vi "tryRead.vi"(8 "error in (no error)":errorcluster, 11 "M1M3SAL in":refnum<class "M1M3SAL.lvclass">) -> (0 "error out":errorcluster, 1 "Timeout":bool, 2 "Message":T1, 3 "M1M3SAL out":refnum<class "M1M3SAL.lvclass">)   [LabVIEW 2016, in "M1M3SupportCommunicator.lvlib" / "M1M3SAL.lvclass"]
uses:
  M1M3SAL.lvclass
  DataTypes/Message.ctl
  DataTypes/MessageHeader.ctl
  DataTypes/MessageTypes.ctl
  DataTypes/MessageTopics.ctl
  M1M3SupportCommunicator.lvlib
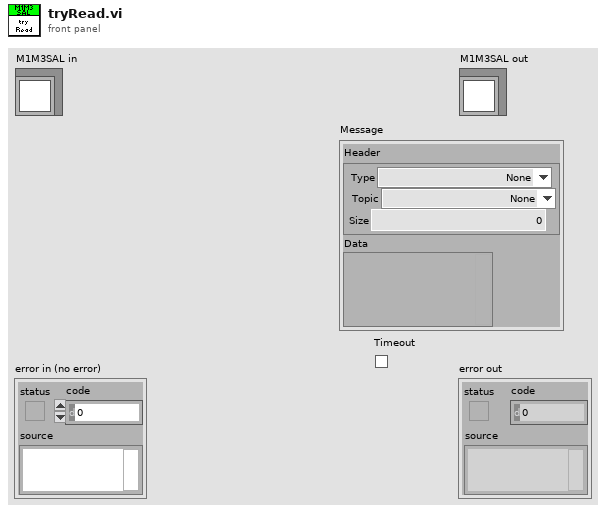
[diagram p1: front panel]
types:
  T1 = typedef "M1M3SupportCommunicator.lvlib/Message.ctl" = cluster{"Header":T2, "Data":variant}
  T2 = typedef "M1M3SupportCommunicator.lvlib/MessageHeader.ctl" = cluster{"Type":T3, "Topic":T4, "Size":i32}
  T3 = typedef "M1M3SupportCommunicator.lvlib/MessageTypes.ctl" = enum8{"None", "PutSample", "GetNextSample", "LogEvent", "GetEvent", "IssueCommand", "CommandId", "WaitForCompletion", "AcceptCommand", "AckCommand"}
  T4 = typedef "M1M3SupportCommunicator.lvlib/MessageTopics.ctl" = enum8{"None", "ForceActuatorData", "MirrorForceData", "HardpointData", "AirData", "DynamicData", "FPGAData", "IMSData", "ForceActuatorStatus", "ElevationData", "HardpointStatus", "HardpointActuatorChase", "AirStatus", "ForceActuatorSafetyChecks", "ForceActuatorTest", "ActuatorBroadcastCounter", "StatusChecks", "CellChecks", "HardpointActuatorBreakaway", "RaiseMirrorComplete", "ILCCommunication", "ElevationAngleChecks", "DetailedState", "ServoLoops", "ForceActuatorInfo", "LowerMirrorComplete", "HardpointActuatorInfo", "SettingsApplied", "ErrorCode", "StartupChecks", "SummaryState", "SettingVersions", "ActuatorTestStatus", "AppliedSettingsMatchStart", "Enable", "EnterMaintenance", "Standby", "AbortLowerM1M3", "ApplyAberrationByForces", "ApplyAOSCorrectionByBendingModes", "ClearAOSCorrection", "Start", "RaiseM1M3", "TestForceActuator", "LowerM1M3", "ApplyAOSCorrectionByForces", "Disable", "ApplyAberationByBendingMode", "TestHardpoint", "ManipulateM1M3", "ClearAberration", "Exit", "TestAir", "AbortRaiseM1M3", "MoveHardpointActuators", "ExitMaintenance", "Shutdown"}
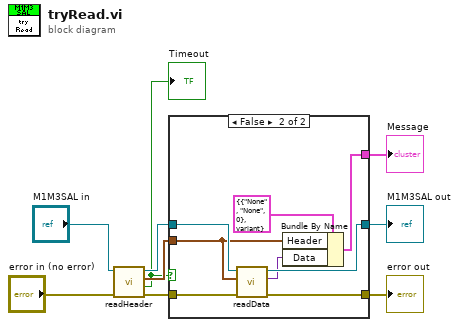
[diagram p0: block diagram]
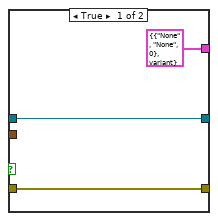
[diagram p2: hidden frame]
diagram:
  n1 = call "readHeader.vi"("error in (no error)"="error in (no error)", "M1M3SAL in"="M1M3SAL in") -> ("error out"=w5:errorcluster, "Timeout"=w1:bool, "Header"=w3:T2, "M1M3SAL out"=w8:refnum<class "M1M3SAL.lvclass">)  [unwired: 6 in]
  "Timeout" <- w1
  n2 = case shown="False" w1 {
    tunnel: w8 -> [w10 w20]
    tunnel: [w10 w19] -> w7
    tunnel: w5 -> [w11 w18]
    tunnel: [w11 w17] -> w4
    tunnel: w3 -> [_ w15]
    tunnel: [T1 {"Header"={"Type"=enum."None", "Topic"=enum."None", "Size"=0}, "Data"=variant} ("Message") w13] -> w2
    frame True {
    }
    frame False {
      n3 = call "readData.vi"("error in (no error)"=w18, "Header"=w15, "M1M3SAL in"=w20) -> ("error out"=w17:errorcluster, "Data"=w14:variant, "M1M3SAL out"=w19:refnum<class "M1M3SAL.lvclass">)  [unwired: 6 in]
      n4 = Bundle By Name(cluster=T1 {"Header"={"Type"=enum."None", "Topic"=enum."None", "Size"=0}, "Data"=variant} ("Message"), "Header"=w15, "Data"=w14) -> (w13:T1)
    }
  }
  "error out" <- w4
  "M1M3SAL out" <- w7
  "Message" <- w2
